vi "Abort.vi"(0 "device session in":refnum<class "Device Session.lvclass">, 11 "error in":errorcluster) -> (4 "device session out":refnum<class "Device Session.lvclass">, 15 "error out":errorcluster)   [LabVIEW 2015, in "Device Session.lvclass"]
doc: "Stops the signal or record acquisition on the FPGA. The acquisition stops immediately. Therefore, after you call the Abort VI, the most recently acquired record may be incomplete. After stopping the acquisition, the Abort VI retains the acquisition state to enable you to fetch previously acquired records even after you abort the acquisition. You cannot use this VI to abort a pending fetch.\n\n<B>Input Parameters</B>\n\n<B>device session in</B> is a reference to the session containing sessions to all instrument design libraries used in this sample project. This parameter is obtained from the 'Open Session' VI.\n\n<B>error in</B> describes error conditions that occur before this node runs. This input provides standard 'error in' functionality.\n\n<B>Output Parameters</B>\n\n<B>device session out</B> passes a reference to the session to the next VI.\n\n<B>error out</B> contains error information. This output provides standard 'error out' functionality."
uses:
  Device Session.lvclass
  Device Session.lvclass/Device Session.ctl
  FPGA Refnum.ctl
  <vilib>/Utility/error.llb/Error Cluster From Error Code.vi
  <vilib>/rvi/errors/niLvFpgaAdjustHostInterfaceError.vi
  <vilib>/rvi/interface/nirviReadWriteControl/nirviReadWriteControl.xnode
  NiFpgaLv.dll
  <vilib>/rvi/interface/Simulation/niFpgaSimulationCallBeginRW.vi
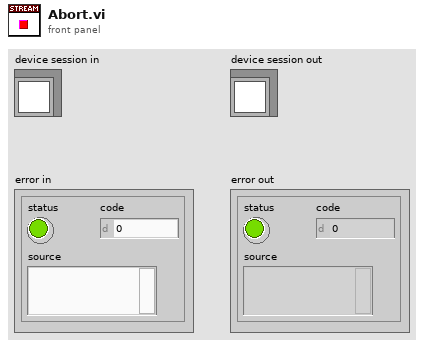
[diagram p1: front panel]
types:
  T1 = typedef "Device Session.lvclass/FPGA Refnum.ctl" = refnum<k20>
  T2 = typedef "Device Session.lvclass/Device Session Object.ctl" = cluster{"ni5171R FPGA Reference":T1, "niHSAI config":refnum<class "niHSAI Config v1 Host.lvclass">, "configured scaling coefficients":cluster{"gain":dbl, "offset":dbl}[], "number of channels to stream":u8, "selected acq channels":bool[], "number of channels":u32, "actual channel configuration":T3[], "configured channels":bool[], "sample clock rate (Hz)":dbl}
  T3 = typedef "niHSAI Types v1 Host.lvlib/Channel Configuration.ctl" = cluster{"channel":u32, "coupling":T4, "impedance":T5, "bandwidth":T6, "vertical range":dbl, "vertical offset":dbl}
  T4 = typedef "niHSAI Types v1 Host.lvlib/Coupling.ctl" = enum8{"Default", "DC", "AC"}
  T5 = typedef "niHSAI Types v1 Host.lvlib/Impedance.ctl" = enum8{"Default", "1 mega ohm", "50 ohm"}
  T6 = typedef "niHSAI Types v1 Host.lvlib/Bandwidth.ctl" = enum8{"Default", "Full Bandwidth", "Anti-alias Filter"}
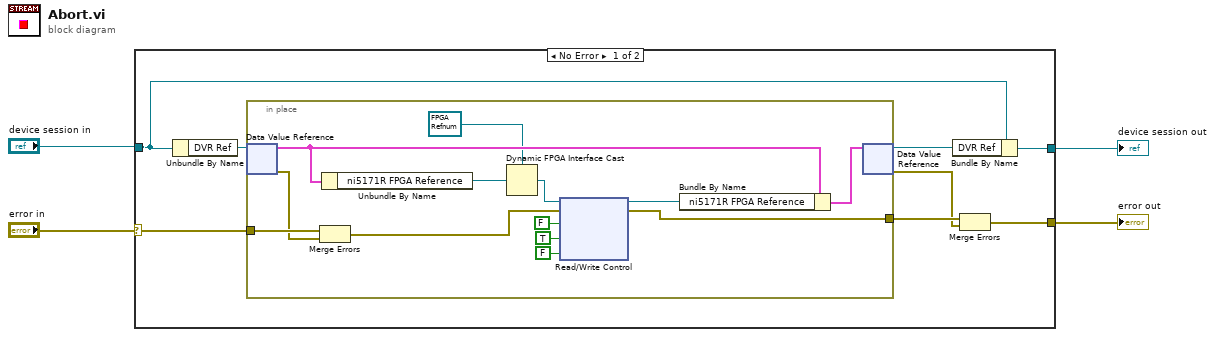
[diagram p0: block diagram]
diagram:
  n1 = case shown="No Error" "error in" {
    selector: "error in" -> [w12 w27]
    tunnel: [w7 w27] -> w3
    tunnel: "device session in" -> [w9 w26]
    tunnel: [w8 w26] -> w1
    frame No Error {
      n2 = Unbundle By Name(w9) -> ("DVR Ref"=w11:refnum<data-value>)
      n3 = in-place {
        in-place-border: w12 -> [w18]
        in-place-border: [w21] -> w6
        n4 = in-place-dvr #1(w11) -> (w25:T2, w17:errorcluster)
        n5 = Merge Errors(w18, w17) -> (w22:errorcluster)
        n6 = Unbundle By Name(w25) -> ("ni5171R FPGA Reference"=w16:T1)
        n7 = Dynamic FPGA Interface Cast(Session In=T1 refnum ("FPGA Interface"), Type=w16) -> (Session Out=w15:T1)
        n8 = xnode "Read/Write Control"("FPGA VI Reference In"=w15, "error in"=w22, "acq.abort"=FALSE ("acq.enabled"), "acq.abort"=TRUE, "acq.abort"=FALSE) -> ("FPGA VI Reference Out"=w23:T1, "error out"=w21:errorcluster)
        n9 = Bundle By Name(cluster=w25, "ni5171R FPGA Reference"=w23) -> (w24:T2)
        n10 = in-place-dvr #1(w24) -> (w10:refnum<data-value>, w5:errorcluster)
      }
      n11 = Bundle By Name(cluster=w9, "DVR Ref"=w10) -> (w8:refnum<class "Device Session.lvclass">)
      n12 = Merge Errors(w6, w5) -> (w7:errorcluster)
    }
    frame Error {
    }
  }
  "error out" <- w3
  "device session out" <- w1
